vi "Write Log Header.vi"(8 "error in (no error)":errorcluster, 11 "Model in":refnum<class "Model.lvclass">) -> (0 "error out":errorcluster, 3 "Model out":refnum<class "Model.lvclass">)   [LabVIEW 2016, in "Model.lvclass"]
uses:
  Model.lvclass
  Model.lvclass/Model.ctl
  Test Log/Test Log/Test Log.lvclass
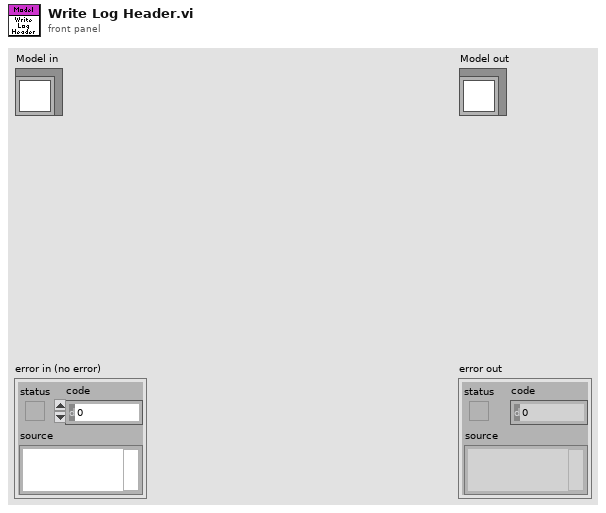
[diagram p1: front panel]
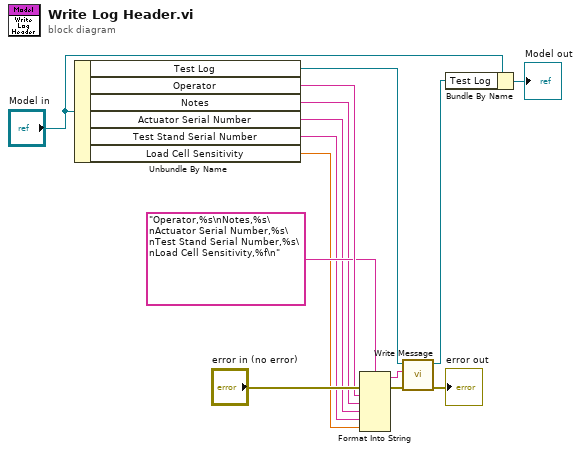
[diagram p0: block diagram]
diagram:
  n1 = Unbundle By Name("Model in") -> ("Test Log"=w13:refnum<class "Test Log.lvclass">, "Operator"=w6:string, "Notes"=w4:string, "Actuator Serial Number"=w3:string, "Test Stand Serial Number"=w2:string, "Load Cell Sensitivity"=w1:dbl)
  n2 = Format Into String(format string="Operator,%s\nNotes,%s\nActuator Serial Number,%s\nTest Stand Serial Number,%s\nLoad Cell Sensitivity,%f\n", error in="error in (no error)", w6, w4, w3, w2, w1) -> (resulting string=w14:string, error out=w10:errorcluster)  [unwired: 1 in]
  n3 = call-dynamic "Write Message.vi"("error in (no error)"=w10, "Message"=w14, "Test Log in"=w13) -> ("error out"=→"error out":errorcluster, "Test Log out"=w12:refnum<class "Test Log.lvclass">)  [unwired: 7 in]
  n4 = Bundle By Name(cluster="Model in", "Test Log"=w12) -> (→"Model out":refnum<class "Model.lvclass">)
